vi "Request Synchronous Variant.vi"(6 "Ignore Past Updates? (F)":bool, 7 "Timeout In ms (-1)":i32=-1, 8 "error in (no error)":errorcluster, 9 "Type":variant, 10 "Datum Name":string, 11 "IObserver In":refnum<class "IObserver.lvclass">) -> (0 "error out":errorcluster, 1 "timed out?":bool, 2 "Data":variant, 4 "Publication Time":timestamp)   [LabVIEW 2017, in "IObserver.lvlib" / "IObserver.lvclass"]
doc: "DEPRECATED by Request Synchronous Data.vim"
uses:
  IObserver.lvclass
  IObserver.lvclass/IObserver.ctl
  SubscriptionPolicy/OneShotSubscription/OneShotSubscription.lvclass/OneShotSubscription.ctl
  gpm_packages/@cs/transport/Source/Concrete/NotifierTransport/NotifierTransport.lvclass/NotifierTransport.ctl
  IMediator/SubscriptionRequest/SubscriptionRequest.lvclass/SubscriptionRequest.ctl
  AbstractMessages/PreAddressedMsg/PreAddressedMsg.lvclass/PreAddressedMsg.ctl
  IMediator/IMediator Messages/Subscribe Msg/Subscribe Msg.lvclass/Subscribe Msg.ctl
  <vilib>/ActorFramework/Message Enqueuer/Message Enqueuer.lvclass/Message Enqueuer.ctl
  <vilib>/ActorFramework/Message Enqueuer/Enqueue.vi
  AbstractMessages/PreAddressedMsg/Read Return Address.vi
  gpm_packages/@cs/transport/Source/Concrete/NotifierTransport/NotifierTransport.lvclass
  C:/Git/mva-framework/gpm_packages/@cs/transport/Source/ITransport/ITransport.lvclass
  SubscriptionPolicy/OneShotSubscription/OneShotSubscription.lvclass
  C:/Git/mva-framework/Source/Framework/IMediator/ISubscriptionPolicy/ISubscriptionPolicy.lvclass
  IMediator/IMediator Messages/Subscribe Msg/Subscribe Msg.lvclass
  C:/Git/mva-framework/Source/Framework/AbstractMessages/PreAddressedMsg/PreAddressedMsg.lvclass
  C:/Program Files (x86)/National Instruments/LabVIEW 2017/vi.lib/ActorFramework/Message/Message.lvclass
  <vilib>/Utility/error.llb/Error Cluster From Error Code.vi
  <vilib>/ActorFramework/Message Priority Queue/Priority Enqueue.vi
  IMediator/SubscriptionRequest/SubscriptionRequest.lvclass
  IMediator/ISubscriptionPolicy/ISubscriptionPolicy.lvclass
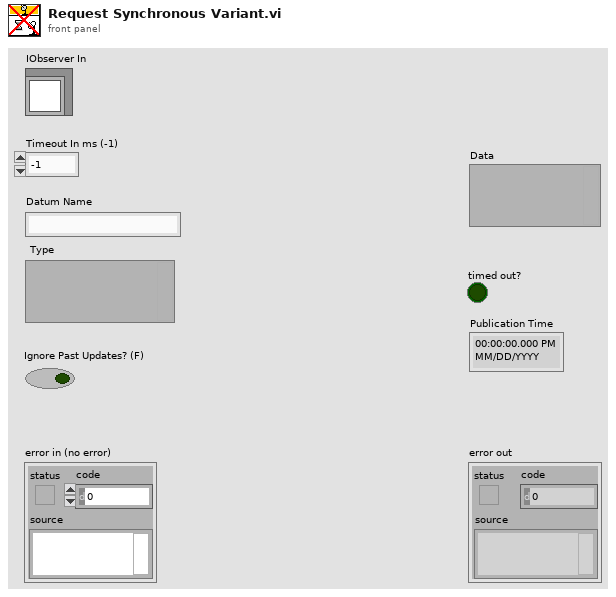
[diagram p1: front panel]
types:
  T1 = typedef "IMediator.lvlib/ISubscriptionPolicy.lvclass/ISubscriptionPolicy Reference.ctl" = refnum<data-value>
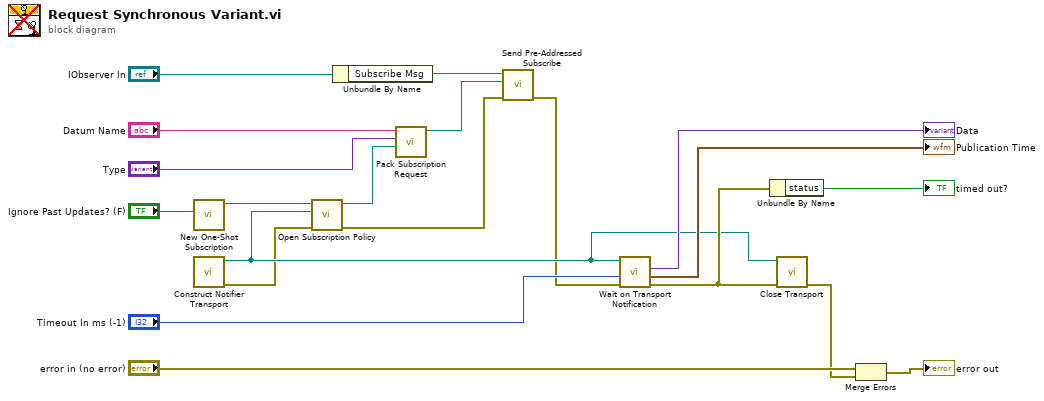
[diagram p0: block diagram]
diagram:
  n1 = call "New One-Shot Subscription.vi"("Ignore Past Updates? (F)"="Ignore Past Updates? (F)") -> ("OneShotSubscription Out"=w17:refnum<class "OneShotSubscription.lvclass">)  [unwired: 10 in]
  n2 = call "Construct Notifier Transport.vi"() -> ("error out"=w3:errorcluster, "NotifierTransport"=w4:refnum<class "NotifierTransport.lvclass">)  [unwired: 10 in]
  n3 = call "Open Subscription Policy.vi"("error in (no error)"=w3, "Transport"=w4, "SubscriptionPolicy"=w17) -> ("error out"=w2:errorcluster, "Subscription Policy"=w5:T1)  [unwired: 7 in]
  n4 = Unbundle By Name("IObserver In") -> ("Subscribe Msg"=w14:refnum<class "Subscribe Msg.lvclass">)
  n5 = call "Pack Subscription Request.vi"("Subscription Policy"=w5, "Type"="Type", "Datum Name"="Datum Name") -> ("SubscriptionRequest"=w13:refnum<class "SubscriptionRequest.lvclass">)  [unwired: 8 in]
  n6 = call "Send Pre-Addressed Subscribe.vi"("error in (no error)"=w2, "Subscription Request"=w13, "Subscribe Msg"=w14) -> ("error out"=w1:errorcluster)  [unwired: 8 in]
  n7 = call "Wait on Transport Notification.vi"("error in (no error)"=w1, "Timeout In ms (-1)"="Timeout In ms (-1)", "NotifierTransport"=w4) -> ("error out"=w6:errorcluster, "Publication Time"=→"Publication Time":timestamp, "Data"=→"Data":variant)  [unwired: 6 in]
  n8 = Unbundle By Name(w6) -> ("status"=→"timed out?":bool)
  n9 = call-dynamic "Close Transport.vi"("error in (no error)"=w6, "NotifierTransport"=w4) -> ("error out"=w8:errorcluster)  [unwired: 9 in]
  n10 = Merge Errors("error in (no error)", w8) -> (→"error out":errorcluster)
